vi "第一回合上位机.vi"() -> ()   [LabVIEW 2016]
uses:
  Hokuyo URG Series/Public/Initialize-Standard.vi
  Hokuyo URG Series/Hokuyo URG Series.lvlib
panel:
  out "XY图":cluster{"X":dbl[], "Y":dbl[]}[](graph)
  in  "数据输入 2":string="0000000000003"
  out "流程":bool
  in  "字符串":string
  in  "角度":dbl
  in  "投球y":dbl
  in  "投球x":dbl
  in  "停止距离":dbl
  out "数据输出":string
  out "输出角度":dbl
  out "输出判断位":i32
  out "输出y":i32
  out "输出x":i32
  out "枚举":T1
  in  "分割距离阈值":dbl=2500.0 format="%#_13g"
  in  "最少用到的点个数":i32=10
  in  "半径下限":dbl(slide)=68.44547563805105 scale=0.0..500.0
  in  "半径上限":dbl(slide)=115.66820276497695 scale=100.0..500.0
  in  "拟合度阈值":dbl=0.03
  in  "Encoding Width":u16(ring)=3 items=["2 Byte"=2, "3 Byte"=3]
  in  "Cluster Count":dbl=1.0
  in  "Start Point":dbl=-60.0
  in  "End Point":dbl=60.0
  in  "Protocol":u32(ring)=2 items=["Convert to Latest", "SCIP 1.1", "SCIP 2.0"]
  in  "ID Query?":bool=TRUE
  in  "Checksum":bool
  in  "VISA resource name":refnum<visa-resource-name>
  in  "停止":bool
  in  "写入的字节":i32
  in  "数据输入":string="12345678912345"
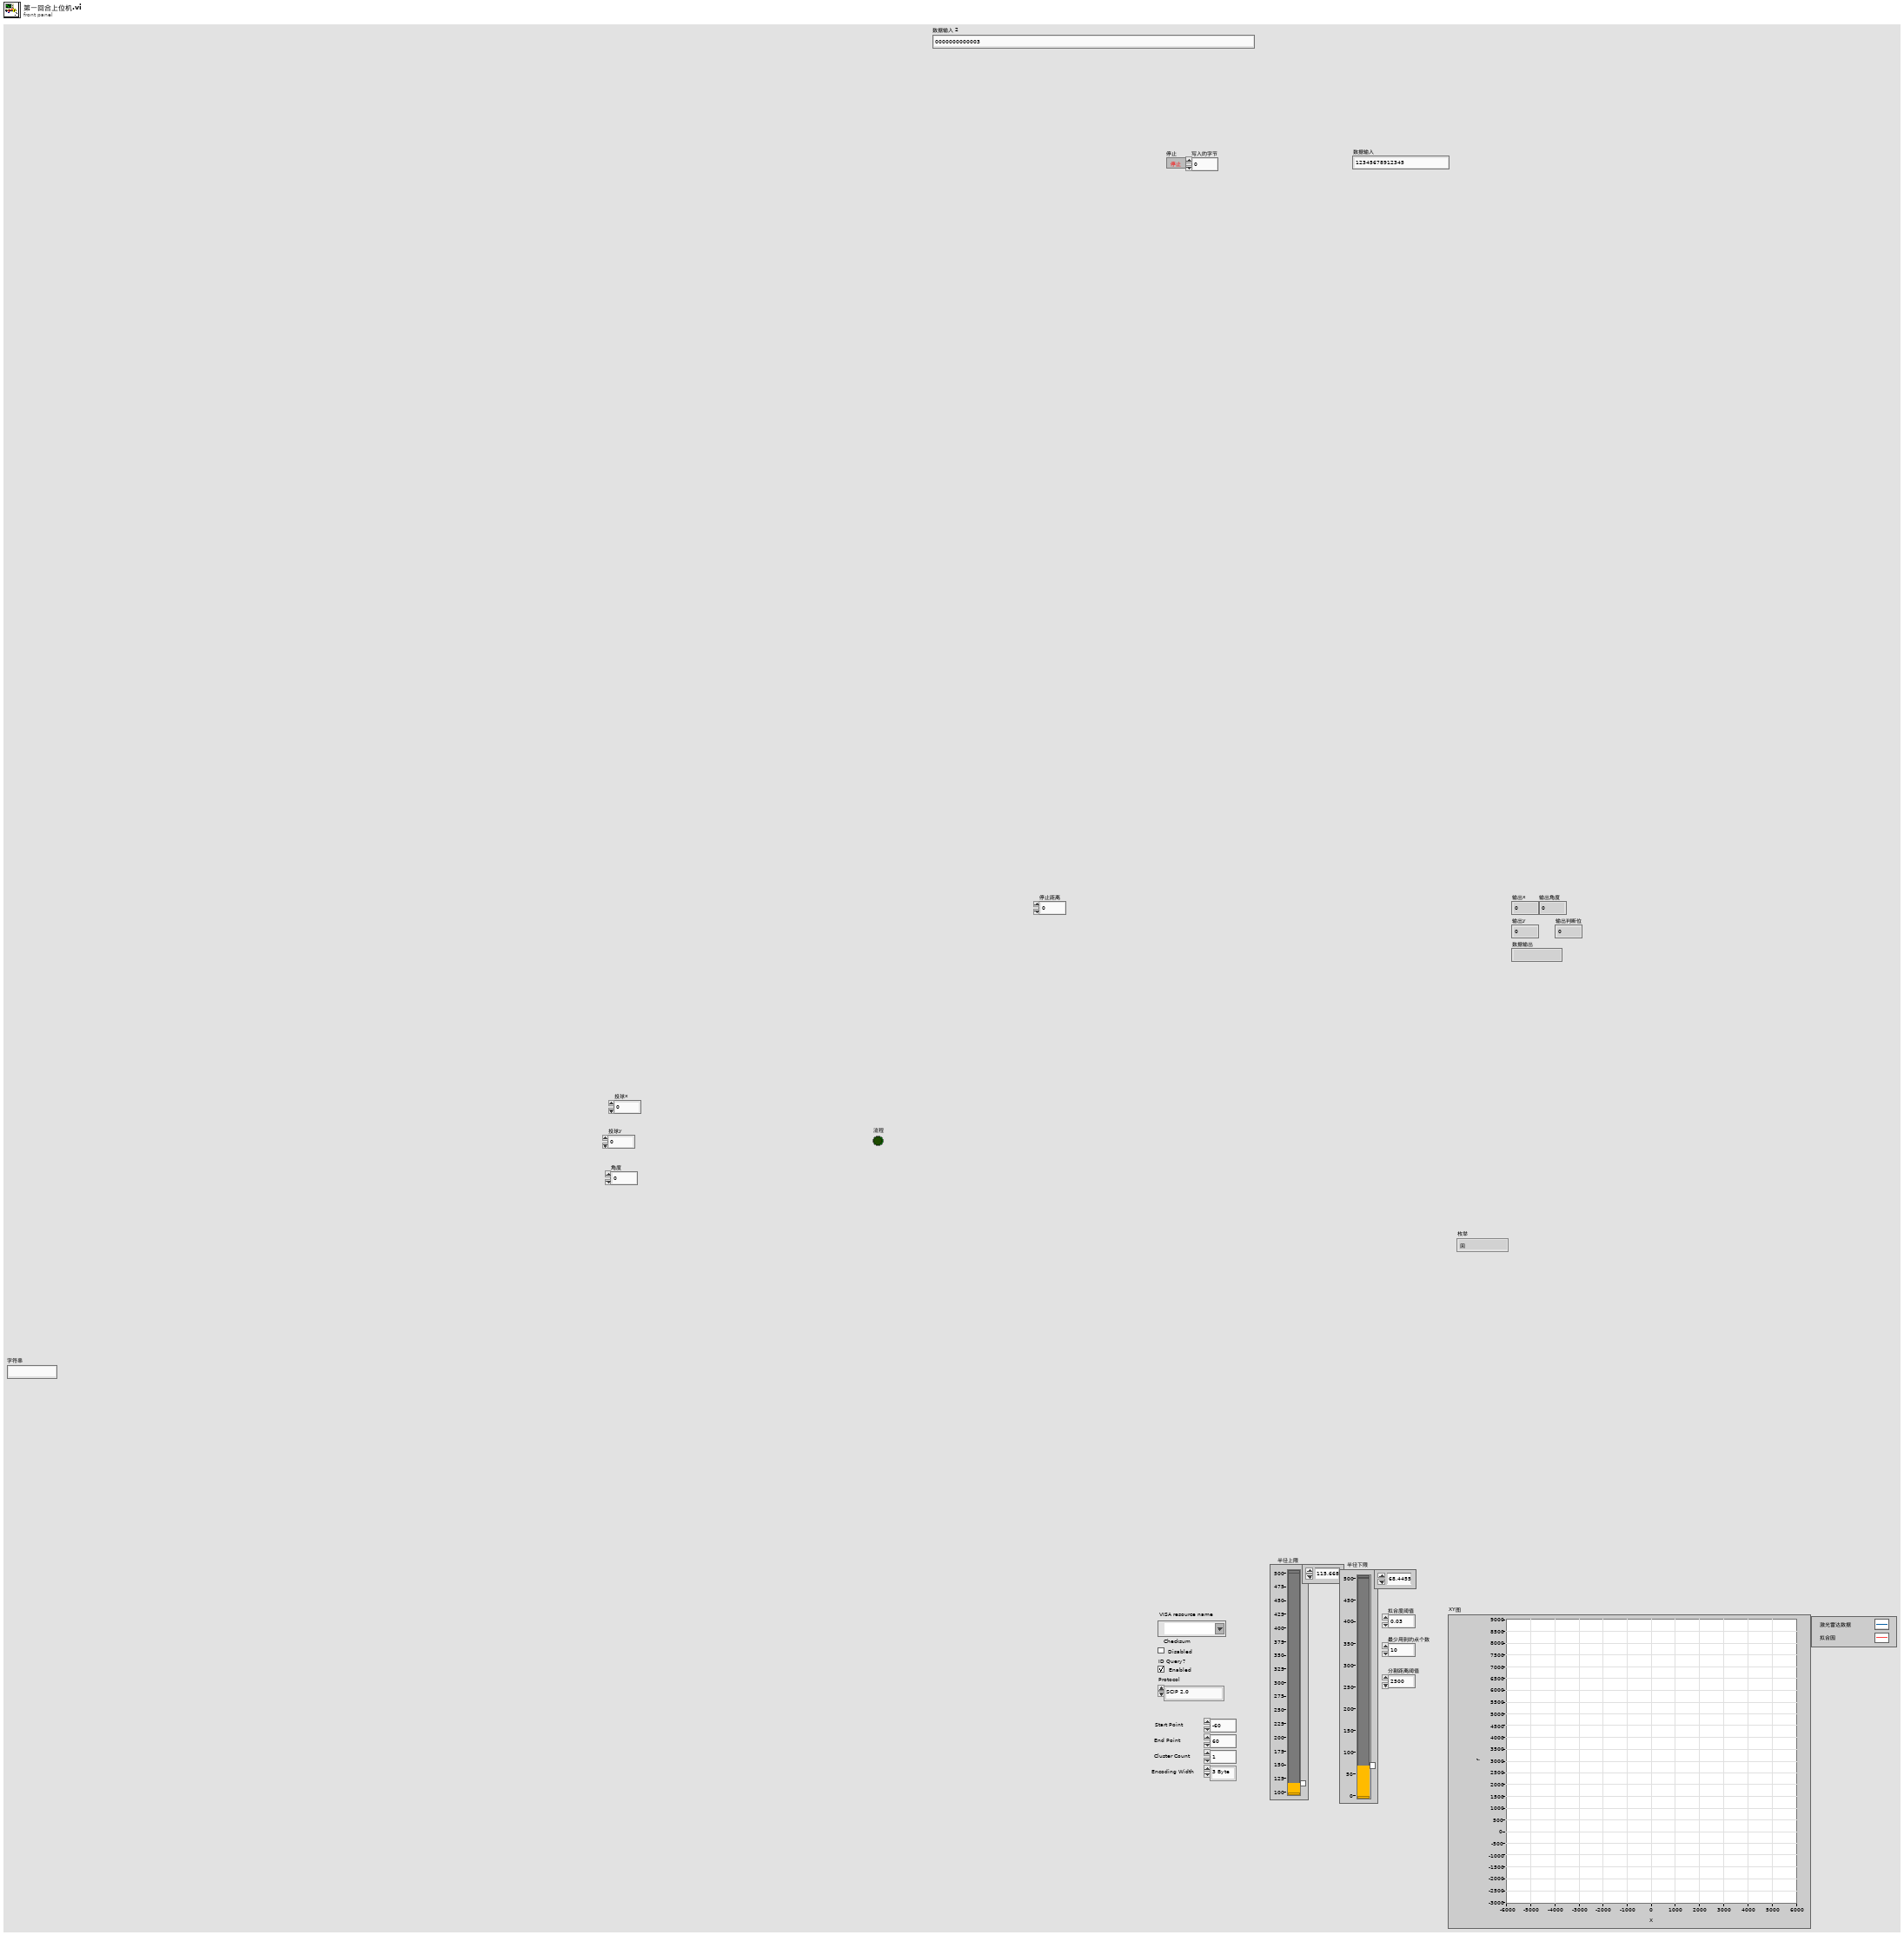
[diagram p1: front panel]
types:
  T1 = typedef "第一回合状态.ctl" = enum16{"回", "前进", "搜索球", "旋转", "铲球", "投球"}
  T2 = cluster{"方差（越小越好）":dbl, "距离（mm）":dbl, "角度":dbl, "半径":dbl, "有效点个数":i32, "弧的张角":dbl}[]
  T3 = cluster{"方差（越小越好）":dbl, "距离（mm）":dbl, "角度":dbl, "半径":dbl, "有效点个数":i32, "弧的张角":dbl}
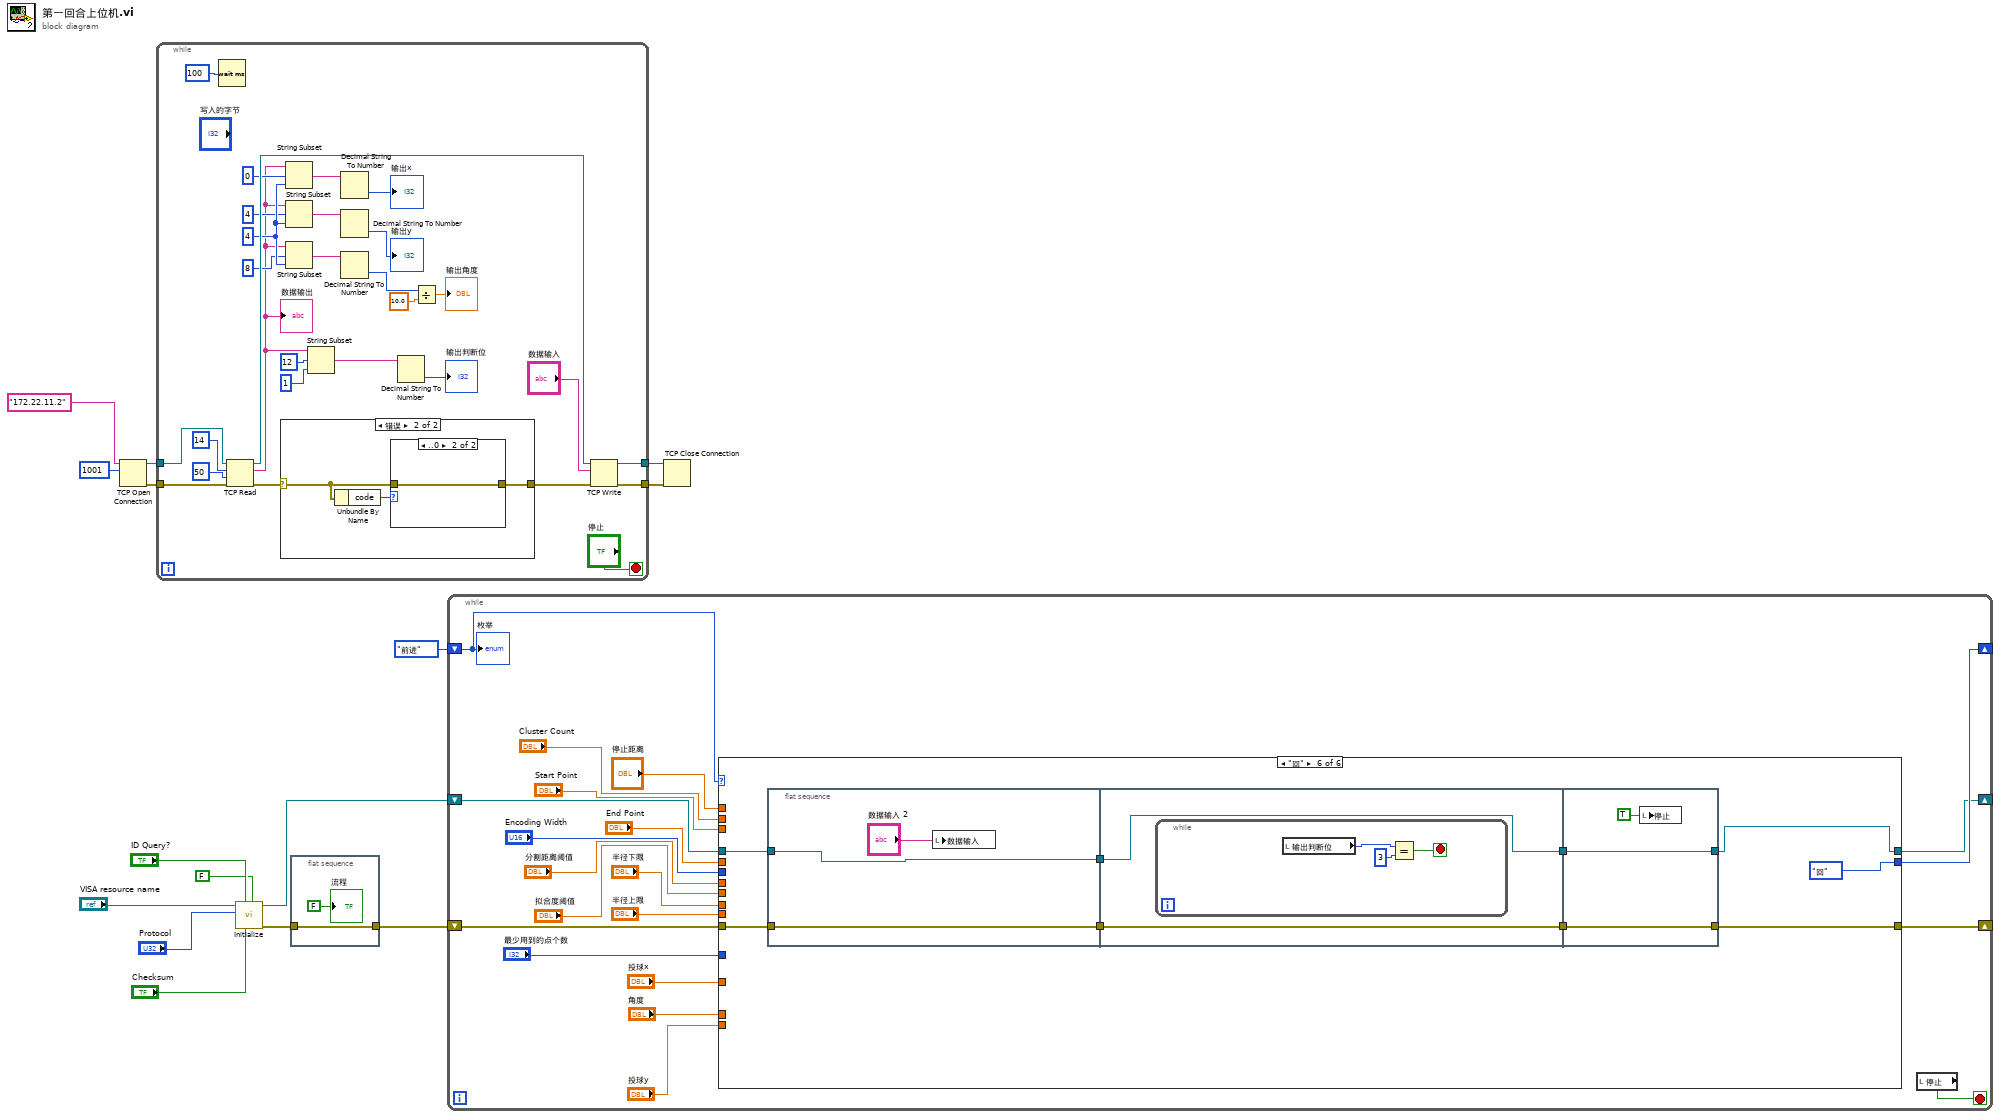
[diagram p0: block diagram]
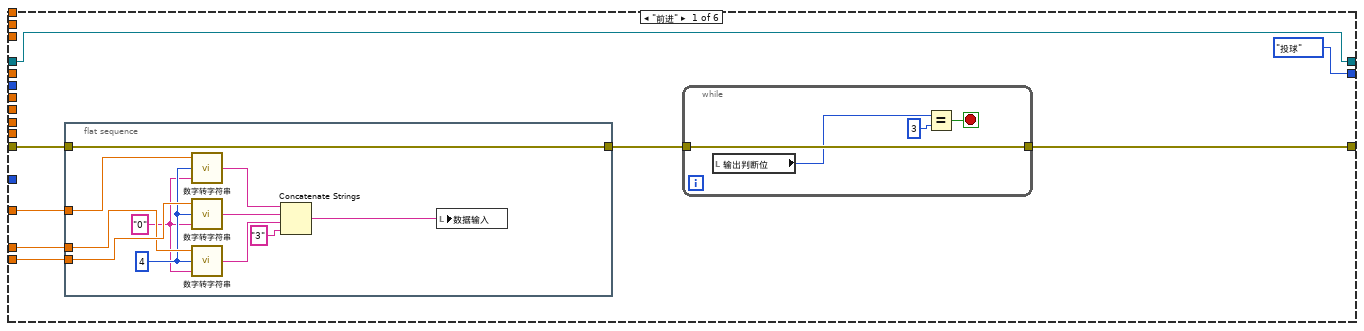
[diagram p2: hidden frame]
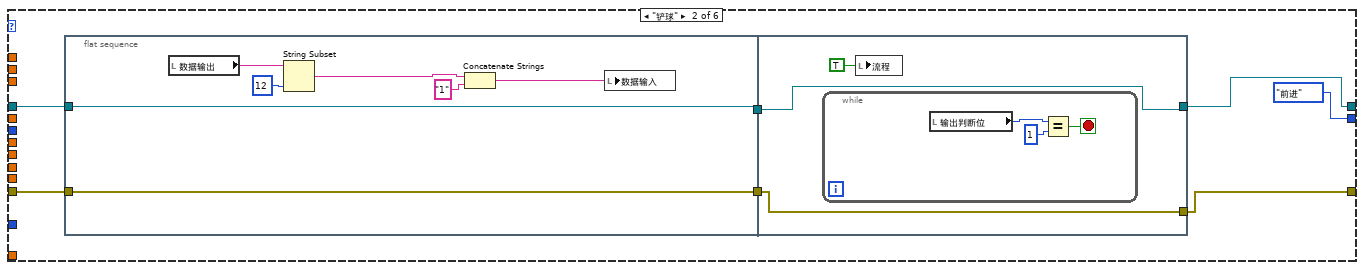
[diagram p3: hidden frame]
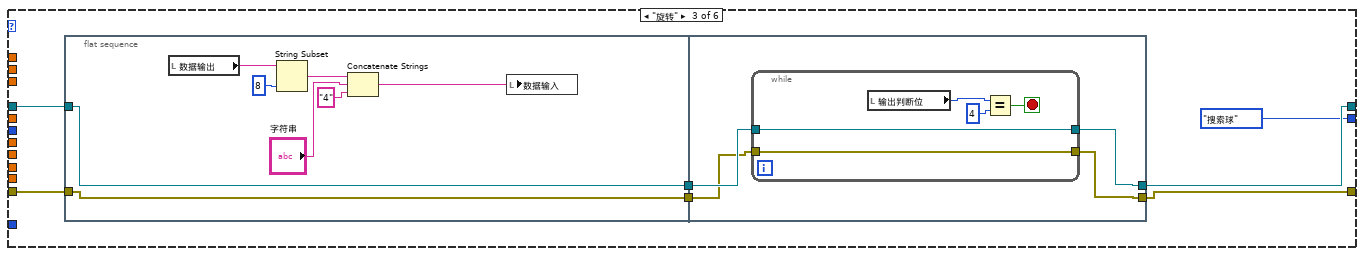
[diagram p4: hidden frame]
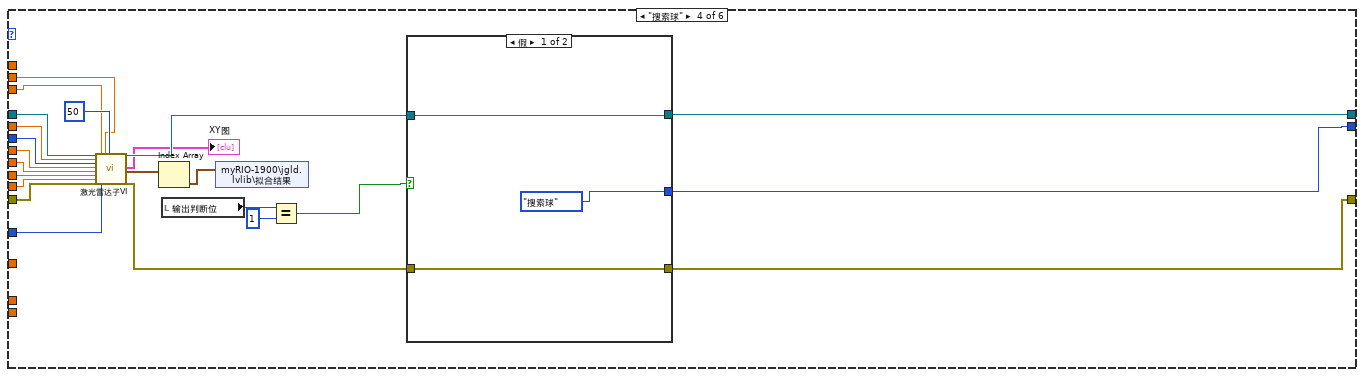
[diagram p5: hidden frame]
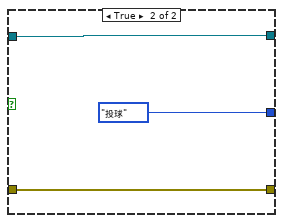
[diagram p6: hidden frame]
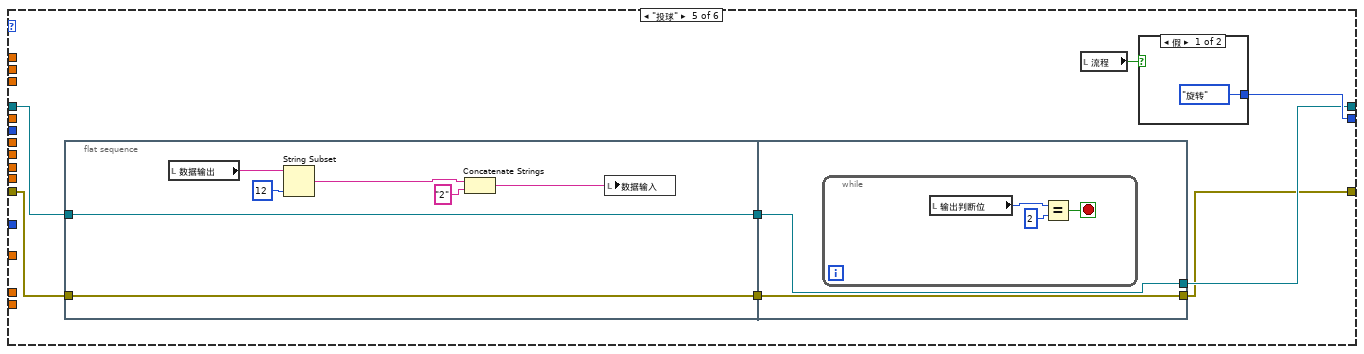
[diagram p7: hidden frame]
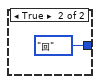
[diagram p8: hidden frame]
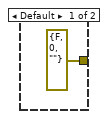
[diagram p10: hidden frame]
diagram:
  n1 = TCP Open Connection(address="172.22.11.2" ("地址"), remote port or service name=u16 1001 ("远程端口或服务名称")) -> (connection ID=w15:refnum<k5>, error out=w14:errorcluster)  [unwired: 3 in]
  n2 = while {
    tunnel: w15 -> [w44]
    tunnel: w14 -> [w43]
    tunnel: [w37] -> w13
    tunnel: [w35] -> w12
    stop <- "停止" stop-if-true
    w31 = 4 ("长度（剩余）")
    n3 = Wait (ms)(milliseconds to wait=100) -> ()  [unwired: 1 out]
    n4 = TCP Read(connection ID=w44, bytes to read=14 ("读取的字节"), error in (no error)=w43, 9:50) -> (connection ID out=w38:refnum<k5>, data out=w26:string, error out=w41:errorcluster)  [unwired: 1 in]
    "数据输出" <- w26
    n5 = case shown="错误" w41 {
      selector: w41 -> [w45 w46]
      tunnel: [w45 w47] -> w36
      frame No Error {
      }
      frame Error {
        n6 = Unbundle By Name(w46) -> ("code"=w48:i32)
        n7 = case shown="..0" w48 {
          tunnel: [errorcluster {"status"=FALSE, "code"=0, "source"=""} ("error IO") w50] -> w47
          tunnel: w46 -> [_ w50]
          frame Default {
          }
          frame ..0 {
          }
        }
      }
    }
    n8 = String Subset(string=w26, offset (0)=0 ("偏移量(0)"), length (rest)=w31) -> (substring=w25:string)
    n9 = String Subset(string=w26, offset (0)=4 ("偏移量(0)"), length (rest)=w31) -> (substring=w24:string)
    n10 = String Subset(string=w26, offset (0)=8 ("偏移量(0)"), length (rest)=w31) -> (substring=w23:string)
    n11 = String Subset(string=w26, offset (0)=12 ("偏移量(0)"), length (rest)=1 ("长度（剩余）")) -> (substring=w22:string)
    n12 = Decimal String To Number(string=w25) -> (number=→"输出x":i32)  [unwired: 2 in, 1 out]
    n13 = Decimal String To Number(string=w24) -> (number=→"输出y":i32)  [unwired: 2 in, 1 out]
    n14 = Decimal String To Number(string=w23) -> (number=w18:i32)  [unwired: 2 in, 1 out]
    n15 = Decimal String To Number(string=w22) -> (number=→"输出判断位":i32)  [unwired: 2 in, 1 out]
    n16 = Divide(x=w18, y=10.0) -> (x/y=→"输出角度":dbl)
    n17 = TCP Write(connection ID=w38, data in="数据输入", error in (no error)=w36) -> (connection ID out=w37:refnum<k5>, error out=w35:errorcluster)  [unwired: 1 in, 1 out]
  }
  n18 = call-poly "Initialize.vi"("Reset? (F: No)"=FALSE ("Reset Instrument (Disabled)"), "Checksum (Disabled)"="Checksum", "ID Query? (Enabled)"="ID Query?", "Protocol (2: SCIP 2.0)"="Protocol", "VISA resource name"="VISA resource name") -> ("error out"=w3:errorcluster, "VISA resource name out"=w5:refnum<visa-resource-name>)  [unwired: 5 in]
  n19 = flat-sequence {
    tunnel: [w51] -> w2
    tunnel: w3 -> [w51]
    frame #0 {
      "流程" <- FALSE ("流程")
    }
  }
  n20 = while {
    shift-right: [w70] -> _
    shift-left: 第一回合状态."前进" -> [w71]
    shift-right: [w69] -> _
    shift-left: w5 -> [w53]
    shift-right: [w68] -> _
    shift-left: w2 -> [w54]
    stop <- w72 stop-if-true
    n21 = case shown="\"回\"" w71 {
      tunnel: [第一回合状态."投球" ("枚举") 第一回合状态."前进" 第一回合状态."搜索球" w143 w176 第一回合状态."回"] -> w70
      tunnel: w53 -> [w80 w102 w122 w162 w175 w199]
      tunnel: w54 -> [w76 w100 w120 w161 w173 w197]
      tunnel: [w80 w101 w121 w148 w174 w198] -> w69
      tunnel: [w74 w99 w117 w150 w172 w196] -> w68
      tunnel: "Cluster Count" -> [_ _ _ w159 _ _]
      tunnel: "Start Point" -> [_ _ _ w158 _ _]
      tunnel: "End Point" -> [_ _ _ w157 _ _]
      tunnel: "Encoding Width" -> [_ _ _ w156 _ _]
      tunnel: "分割距离阈值" -> [_ _ _ w155 _ _]
      tunnel: "拟合度阈值" -> [_ _ _ w154 _ _]
      tunnel: "半径下限" -> [_ _ _ w153 _ _]
      tunnel: "半径上限" -> [_ _ _ w152 _ _]
      tunnel: "最少用到的点个数" -> [_ _ _ w151 _ _]
      tunnel: "停止距离" -> [_ _ _ _ _ _]
      tunnel: "投球x" -> [w79 _ _ _ _ _]
      tunnel: "投球y" -> [w78 _ _ _ _ _]
      tunnel: "角度" -> [w77 _ _ _ _ _]
      frame "前进" {
        n22 = flat-sequence {
          tunnel: w79 -> [w91]
          tunnel: w78 -> [w90]
          tunnel: w77 -> [w89]
          tunnel: w76 -> [w81]
          tunnel: [w81] -> w75
          frame #0 {
            w88 = i16 4 ("宽度")
            w87 = "0" ("填充串")
            n23 = call "数字转字符串.vi"("填充串"=w87, "宽度"=w88, "数字"=w91) -> ("输出"=w86:string)
            n24 = call "数字转字符串.vi"("填充串"=w87, "宽度"=w88, "数字"=w90) -> ("输出"=w85:string)
            n25 = call "数字转字符串.vi"("填充串"=w87, "宽度"=w88, "数字"=w89) -> ("输出"=w84:string)
            n26 = Concatenate Strings(w86, w85, w84, "3" ("字符串")) -> (w82:string)
            n27 = local write "数据输入"(w82) -> ()
          }
        }
        n28 = while {
          tunnel: w75 -> [w93]
          tunnel: [w93] -> w74
          stop <- w94 stop-if-true
          n29 = local read "输出判断位"() -> (w92:i32)
          n30 = Equal?(x=w92, y=3) -> (x = y?=w94:bool)
        }
      }
      frame "铲球" {
        n31 = flat-sequence {
          tunnel: w102 -> [w109]
          tunnel: w100 -> [w108]
          tunnel: [w109] -> w98
          tunnel: [w108] -> w97
          tunnel: [w111] -> w99
          tunnel: [w112] -> w101
          tunnel: w98 -> [w112]
          tunnel: w97 -> [w111]
          frame #0 {
            n32 = local read "数据输出"() -> (w103:string)
            n33 = String Subset(string=w103, length (rest)=12 ("长度（剩余）")) -> (substring=w105:string)  [unwired: 1 in]
            n34 = Concatenate Strings(w105, "1" ("字符串")) -> (w107:string)
            n35 = local write "数据输入"(w107) -> ()
          }
          frame #1 {
            n36 = while {
              stop <- w113 stop-if-true
              n37 = local read "输出判断位"() -> (w115:i32)
              n38 = Equal?(x=w115, y=1) -> (x = y?=w113:bool)
            }
            n39 = local write "流程"(TRUE ("流程")) -> ()
          }
        }
      }
      frame "旋转" {
        n40 = flat-sequence {
          tunnel: w122 -> [w130]
          tunnel: w120 -> [w129]
          tunnel: [w130] -> w119
          tunnel: [w129] -> w118
          tunnel: [w131] -> w117
          tunnel: [w134] -> w121
          tunnel: w119 -> [w133]
          tunnel: w118 -> [w132]
          frame #0 {
            n41 = local read "数据输出"() -> (w123:string)
            n42 = String Subset(string=w123, length (rest)=8 ("长度（剩余）")) -> (substring=w125:string)  [unwired: 1 in]
            n43 = Concatenate Strings(w125, "字符串", "4" ("字符串")) -> (w128:string)
            n44 = local write "数据输入"(w128) -> ()
          }
          frame #1 {
            n45 = while {
              tunnel: [w136] -> w134
              tunnel: w133 -> [w136]
              tunnel: w132 -> [w135]
              tunnel: [w135] -> w131
              stop <- w137 stop-if-true
              n46 = local read "输出判断位"() -> (w139:i32)
              n47 = Equal?(x=w139, y=4) -> (x = y?=w137:bool)
            }
          }
        }
      }
      frame "搜索球" {
        n48 = call "激光雷达子VI.vi"("VISA引用句柄输入"=w162, "End Point"=w157, "Encoding Width"=w156, "分割距离阈值"=w155, "拟合度阈值"=w154, "半径下限"=w153, "半径上限"=w152, "错误输入（无错误）"=w161, "Start Point"=w158, "最少用到的点个数"=w151, "Cluster Count"=w159, "等待时间"=u32 50) -> ("VISA引用句柄输出"=w147:refnum<visa-resource-name>, "绘图信息"=→"XY图":cluster{"X":dbl[], "Y":dbl[]}[], "拟合结果"=w141:T2, "错误输出"=w149:errorcluster)  [unwired: 8 in, 4 out]
        n49 = Index Array(array=w141) -> (element=w142:T3)  [unwired: 1 in]
        n50 = local read "输出判断位"() -> (w146:i32)
        n51 = shared-variable "myRIO-1900\\jgld.lvlib\\拟合结果"(w142) -> ()  [unwired: 1 in, 1 out]
        n52 = Equal?(x=w146, y=1) -> (x = y?=w144:bool)
        n53 = case shown="假" w144 {
          tunnel: [w164 w168] -> w150
          tunnel: w149 -> [w164 w168]
          tunnel: [w165 w167] -> w148
          tunnel: w147 -> [w165 w167]
          tunnel: [第一回合状态."搜索球" 第一回合状态."投球"] -> w143
          frame False {
          }
          frame True {
          }
        }
      }
      frame "投球" {
        n54 = flat-sequence {
          tunnel: w175 -> [w185]
          tunnel: w173 -> [w184]
          tunnel: [w185] -> w171
          tunnel: [w184] -> w170
          tunnel: [w186] -> w172
          tunnel: [w187] -> w174
          tunnel: w171 -> [w187]
          tunnel: w170 -> [w186]
          frame #0 {
            n55 = local read "数据输出"() -> (w179:string)
            n56 = String Subset(string=w179, length (rest)=12 ("长度（剩余）")) -> (substring=w181:string)  [unwired: 1 in]
            n57 = Concatenate Strings(w181, "2" ("字符串")) -> (w183:string)
            n58 = local write "数据输入"(w183) -> ()
          }
          frame #1 {
            n59 = while {
              stop <- w188 stop-if-true
              n60 = local read "输出判断位"() -> (w190:i32)
              n61 = Equal?(x=w190, y=2) -> (x = y?=w188:bool)
            }
          }
        }
        n62 = local read "流程"() -> (w169:bool)
        n63 = case shown="假" w169 {
          tunnel: [第一回合状态."旋转" 第一回合状态."回"] -> w176
          frame False {
          }
          frame True {
          }
        }
      }
      frame "回" {
        n64 = flat-sequence {
          tunnel: w199 -> [w202]
          tunnel: w197 -> [w201]
          tunnel: [w202] -> w195
          tunnel: [w201] -> w194
          tunnel: w195 -> [w204]
          tunnel: w194 -> [w203]
          tunnel: [w204] -> w193
          tunnel: [w203] -> w192
          tunnel: [w209] -> w196
          tunnel: [w210] -> w198
          tunnel: w193 -> [w210]
          tunnel: w192 -> [w209]
          frame #0 {
            n65 = local write "数据输入"("数据输入 2") -> ()
          }
          frame #1 {
            n66 = while {
              stop <- w205 stop-if-true
              n67 = local read "输出判断位"() -> (w207:i32)
              n68 = Equal?(x=w207, y=3) -> (x = y?=w205:bool)
            }
          }
          frame #2 {
            n69 = local write "停止"(TRUE ("停止")) -> ()
          }
        }
      }
    }
    n70 = local read "停止"() -> (w72:bool)
    "枚举" <- w71
  }
  n71 = TCP Close Connection(connection ID=w13, error in (no error)=w12) -> ()  [unwired: 1 in, 2 out]
